vi "Msg.Q.Flush.vi"(8 "Error (in)":errorcluster, 11 "Msg.Q.Ref (in)":T1) -> (0 "error out":errorcluster, 3 "Msg.Q.Ref (out)":T1)   [LabVIEW 2023, in "MessagingModule.lvlib"]
doc: "This VI is used to flush a queue message and data."
uses:
  Msg.Q.Ref.ctl
  Msg.Data.ctl
  MessagingModule.lvlib
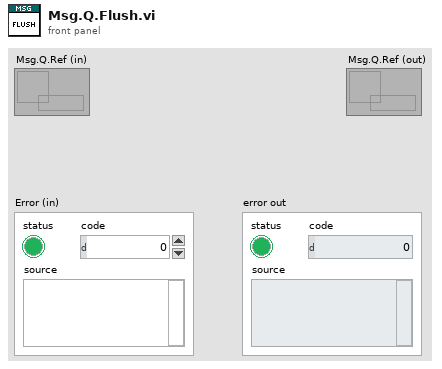
[diagram p1: front panel]
types:
  T1 = typedef "MessagingModule.lvlib/Msg.Q.Ref.ctl" = refnum<queue>
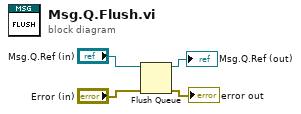
[diagram p0: block diagram]
diagram:
  n1 = Flush Queue(queue="Msg.Q.Ref (in)", error in (no error)="Error (in)") -> (queue out=→"Msg.Q.Ref (out)":T1, error out=→"error out":errorcluster)  [unwired: 1 out]
